vi "A-Scan Processing.vi"(7 "Window":bool=TRUE, 10 "K-Clock":dbl[](array[numeric]), 11 "OCT Signal":dbl[](array[numeric])) -> (3 "A-Scan":dbl[](array[numeric]))   [LabVIEW 2012]
uses:
  <userlib>/Host Processing Library/Windowing/LogFFT with WIndowing.vi
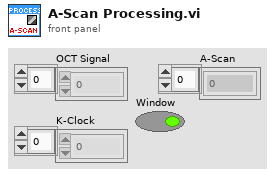
[diagram p1: front panel]
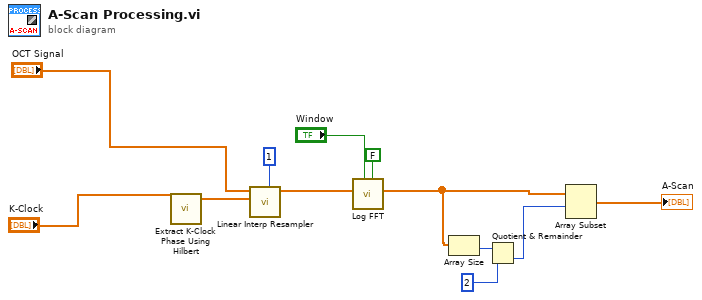
[diagram p0: block diagram]
diagram:
  n1 = call <userlib>:"Extract K-Clock Phase Using Hilbert.vi"("Input Data"="K-Clock") -> ("Hilbert Unwrapped Phase"=w2:dbl[])  [unwired: 10 in]
  n2 = call <userlib>:"Linear Interp Resampler.vi"("interp factor"=1, "K-Data"=w2, "OCT Data"="OCT Signal") -> ("Interpolated Data"=w3:dbl[])  [unwired: 6 in, 2 out]
  n3 = call-poly <userlib>:"Log FFT.vi"("FFT Pad?"=FALSE, "Window"="Window", "FFT {X}"=w3) -> ("Log{Mag(FFT)}"=w9:dbl[])  [unwired: 8 in]
  n4 = Array Size(array=w9) -> (size(s)=w6:i32)
  n5 = Quotient & Remainder(x=w6, y=2) -> (floor(x/y)=w8:i32)  [unwired: 1 out]
  n6 = Array Subset(array=w9, index=w8) -> (→"A-Scan":dbl[])  [unwired: 1 in]
